vi "GUI_TapeDrive.vi"() -> ()   [LabVIEW 2013]
uses:
  Device Driver/TapeDrive/Mode_TypDEf.ctl
  Device Driver/shared/OnOffTypeDef.ctl
  shared programs/GUI_Template/GUI_master/tcp new data cluster.ctl
panel:
  in  "threshold_low::2":dbl=nan caption="threshold low" min=0.0 max=255.0
  in  "threshold_high::2":dbl=0.75 caption="threshold high" min=0.0 max=255.0
  in  "area_min::2":dbl=nan caption="min area" min=10.0 max=50000.0
  in  "area_max::2":dbl=0.75 caption="max area" min=10.0 max=50000.0
  out "cx::2":dbl=nan caption="x" min=0.0 max=0.0
  out "cy::2":dbl=nan caption="y" min=0.0 max=0.0
  out "oldpos::1":dbl=-887.082 caption="position" min=0.0 max=0.0
  out "try::1":dbl=2.0 caption="# of moves\n(scan mode)" min=0.0 max=0.0
  in  "fitnesslimit::2":dbl=0.75 caption="FitnessLimit" min=-100.0 max=1.0
  out "TapeOK":bool
  in  "exposure::3":dbl=0.01 caption="exposure" min=0.0001 max=1.0
  out "image::3":T1(plugin-control) caption="image"
  in  "GUIdevice 3":string="TapeMonitorCamTest"
  out "image::2":T1(plugin-control) caption="Monitor Image (binary)"
  out "particles::2":dbl=nan caption="particles" min=0.0 max=0.0
  out "symmetry::2":dbl=nan caption="Tape Monitor" min=0.0 max=0.0
  out "AreaSymmetry::2":dbl=nan caption="AreaSymmetry" min=0.0 max=0.0
  out "fitness::2":dbl=nan caption="fitness" min=0.0 max=0.0
  in  "TapeOK::2":T2 caption="TapeOK"
  in  "GUIdevice 2":string="TapeMonitorTest"
  in  "resetencoder::1":T2 caption="resetencoder"
  in  "TapeMotor::1":T2 caption="TapeDrive"
  in  "max velocity::1":dbl=5.0 caption="max velocity" min=1.0 max=2000.0
  in  "stepsize::1":dbl=2.0 caption="step size" min=1.0 max=100.0
  in  "timeout::1":dbl=500.0 caption="timeout" min=0.0 max=50000.0
  in  "Step::1":bool caption="Move Tape"
  out "pios chart":dbl(graph)=-887.082 caption="position"
  in  "redratio::1":dbl=1.0 caption="Ratio" min=-2.0 max=2.0
  in  "continious velocity::1":dbl=5.0 caption="continious velocity" min=1.0 max=100.0
  in  "velocity::1":dbl caption="velocity" min=0.0 max=0.0
  in  "Mode::1":T3 caption="Mode"
  in  "direction::1":bool=TRUE caption="Change direction"
  out "position::1":dbl=-887.082 caption="position" min=0.0 max=0.0
  in  "Test Cluster":T4
  out "device status::1":string="Initialized"
  in  "stop":bool
  in  "GUIdevice 1":string="TapeTest"
  # "4"
  # "1"
  # "TapeMotor"
  # "2"
  # "3"
  # "Symmetry"
  # "TapeMonitorCam"
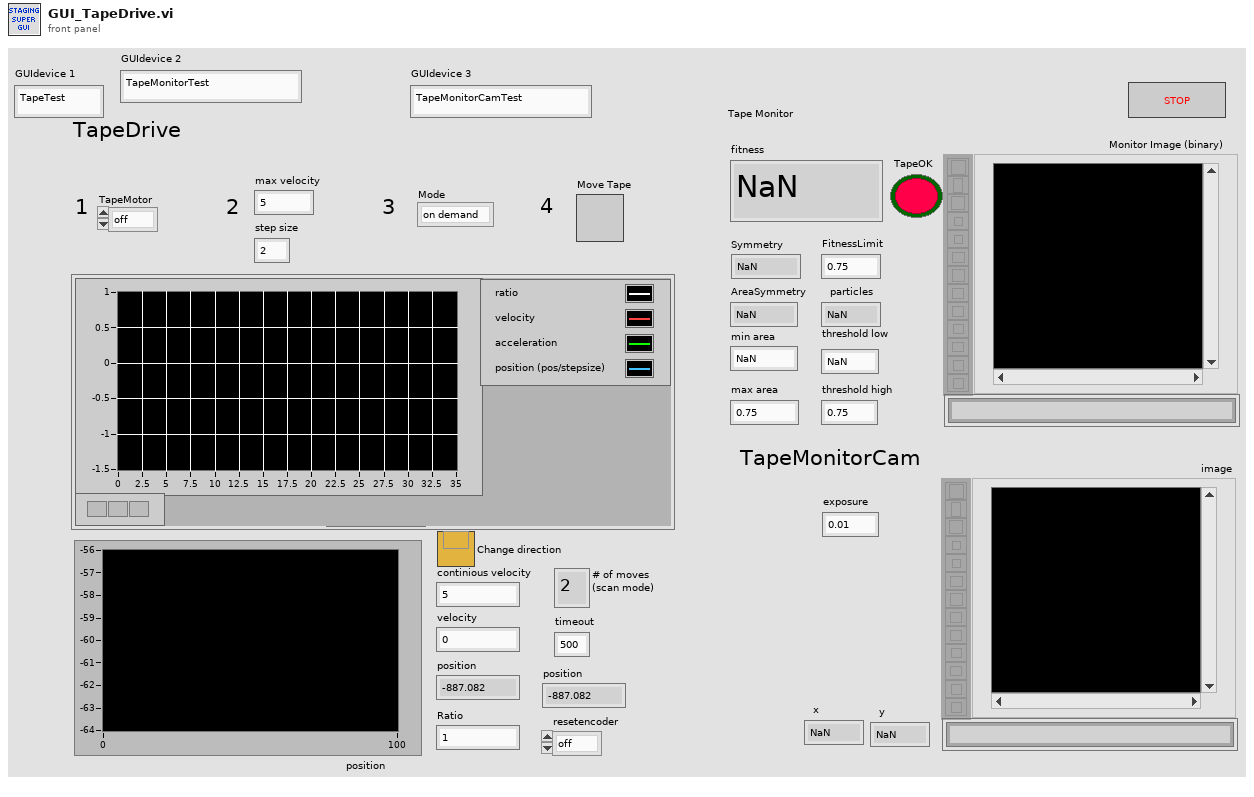
[diagram p1: front panel]
types:
  T1 = typedef "IMAQ Image.ctl" = refnum<image>
  T2 = typedef "OnOffTypeDef.ctl" = enum16{"off", "on"}
  T3 = typedef "Mode_TypDEf.ctl" = enum16{"on demand", "continuous", "scan"}
  T4 = cluster{"Channel::1":enum16{"Channel 0", "Channel 1", "Channel 2", "Channel 3"}, "Trajectory::1":waveform(dbl)[]}
  T5 = typedef "Image Type" = u32
  T6 = typedef "tcp new data cluster.ctl" = cluster{"EventEnum":enum16{"new data", "connection status update"}, "Device name":string}
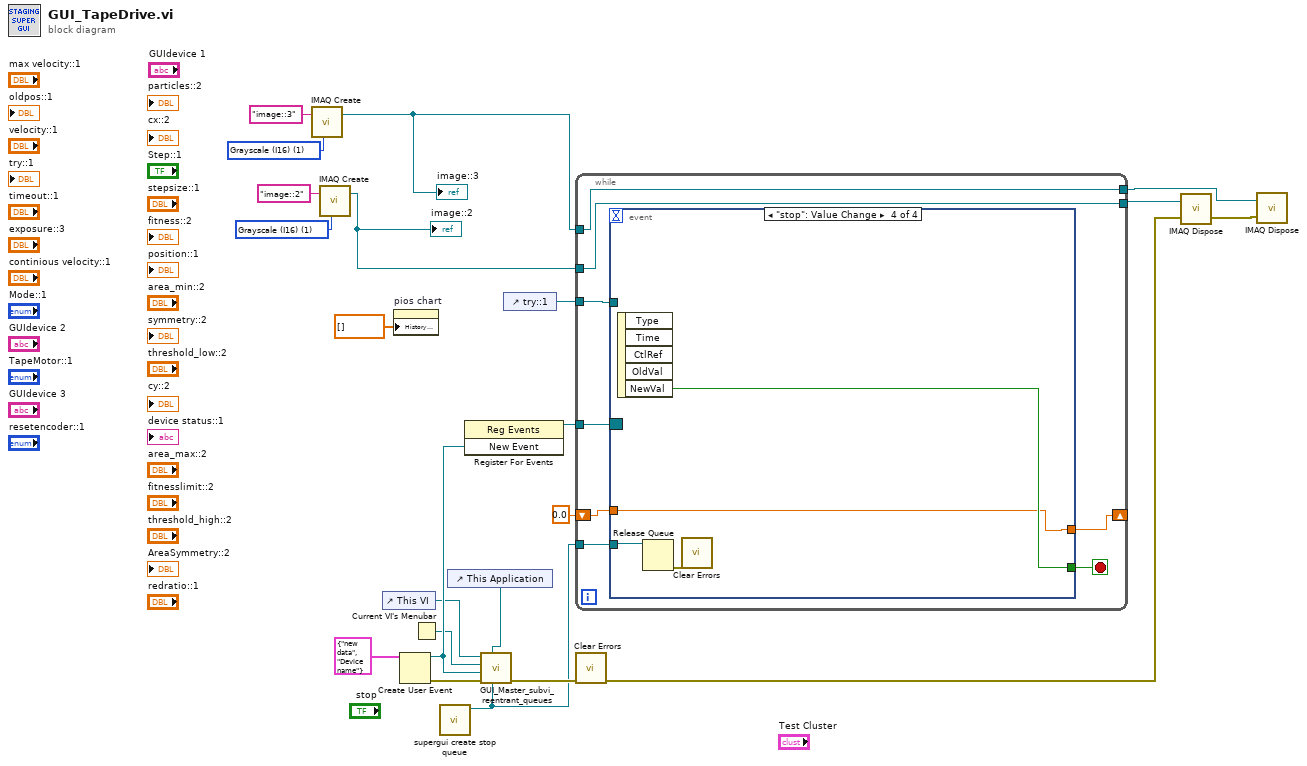
[diagram p0: block diagram]
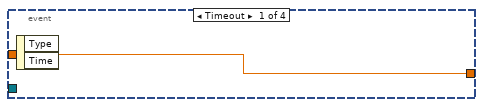
[diagram p2: hidden frame]
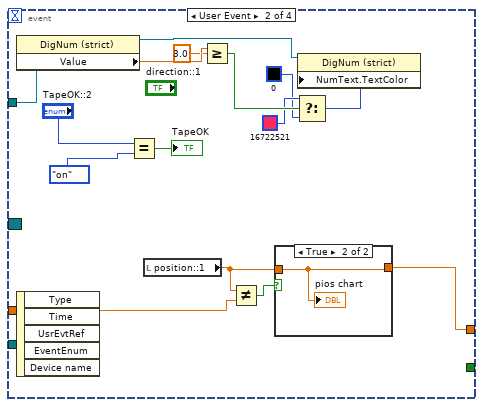
[diagram p3: hidden frame]
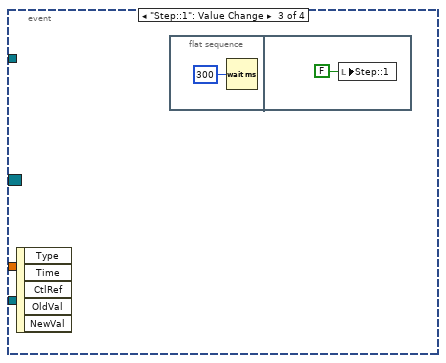
[diagram p5: hidden frame]
diagram:
  w10 = T5 1 items=["Grayscale (U8)", "Grayscale (I16)", "Grayscale (SGL)", "Complex (CSG)", "RGB (U32)", "HSL (U32)", "RGB (U64)", "Grayscale (U16)"] ("Image Type")
  w14 = T5 1 items=["Grayscale (U8)", "Grayscale (I16)", "Grayscale (SGL)", "Complex (CSG)", "RGB (U32)", "HSL (U32)", "RGB (U64)", "Grayscale (U16)"] ("Image Type")
  n1 = call "IMAQ Create"("Image Name"="image::3", "Image Type"=w10) -> ("New Image"=w8:T1)  [unwired: 3 in, 1 out]
  "image::3" <- w8
  n2 = call "IMAQ Create"("Image Name"="image::2", "Image Type"=w14) -> ("New Image"=w13:T1)  [unwired: 3 in, 1 out]
  "image::2" <- w13
  n3 = control-ref of="This VI"() -> (w4:refnum<vi>)
  n4 = property on="pios chart" class="WFChart (strict)"("History Data"=dbl[] []) -> ()  [unwired: 2 in, 2 out]
  n5 = Create User Event(user event datatype=T6 {"EventEnum"=enum."new data", "Device name"="Device name"} ("New Event")) -> (user event=w19:refnum<user-event>, error out=w21:errorcluster)  [unwired: 1 in]
  n6 = Current VI's Menubar() -> (w3:refnum<k9>)
  n7 = call "supergui create stop queue.vi"() -> ("STOP Queue out"=w1:refnum<queue>)  [unwired: 11 in]
  n8 = control-ref of="This Application"() -> (w2:refnum<vi>)
  n9 = register-events(w19) -> (reference out=w18:refnum<event-registration>)  [unwired: 2 in, 1 out]
  n10 = call "GUI_Master_subvi_reentrant_queues.vi"("STOP Queue in"=w1, "This Application"=w2, "error in (no error)"=w21, "tcp data event"=w19, "Caller menu reference"=w3, "Caller VI ref"=w4) -> ("error out"=w20:errorcluster)  [unwired: 5 in]
  n11 = control-ref of="try::1"() -> (w5:refnum<vi>)
  n12 = while {
    tunnel: w18 -> [w30]
    shift-right: [w27] -> _
    shift-left: 0.0 -> [w28]
    tunnel: w13 -> [w26]
    tunnel: [w26] -> w12
    tunnel: w8 -> [w25]
    tunnel: [w25] -> w6
    tunnel: w5 -> [w24]
    tunnel: w1 -> [w23]
    stop <- w29 stop-if-true
    n13 = event shown="[3] \"stop\": Value Change" {
      selector: w30 -> [_ _ _ _]
      dyn-events: _ -> [_ _ _ _]
      timeout: _ -> [_ _ _ _]
      tunnel: [_ _ _ w54] -> w29
      tunnel: w28 -> [w31 w46 _ w53]
      tunnel: [w31 w43 _ w53] -> w27
      tunnel: w24 -> [_ w39 _ _]
      tunnel: w23 -> [_ _ _ w52]
      event Timeout {
        n14 = event-data() -> ()  [unwired: 1 in, 2 out]
      }
      event User Event {
        n15 = property class="DigNum (strict)"(reference=w39) -> (reference out=w36:refnum<vi>, "Value"=w38:dbl)  [unwired: 1 in, 1 out]
        n16 = event-data() -> ()  [unwired: 1 in, 5 out]
        n17 = Equal?(x="TapeOK::2", y=OnOffTypeDef."on" ("TapeOK::2")) -> (x = y?=→"TapeOK":bool)
        n18 = local read "position::1"() -> (w44:dbl)
        n19 = Greater Or Equal?(x=w38, y=3.0) -> (x >= y?=w35:bool)
        n20 = Not Equal?(x=w44, y=w46) -> (x != y?=w45:bool)
        n21 = case shown="True" w45 {
          tunnel: w44 -> [w47 w48]
          tunnel: [w47 w48] -> w43
          frame False {
          }
          frame True {
            "pios chart" <- w48
          }
        }
        n22 = Select(t=u32 16722521, s=w35, f=u32 0) -> (s? t:f=w32:u32)
        n23 = property class="DigNum (strict)"(reference=w36, "NumText.TextColor"=w32) -> ()  [unwired: 1 in, 2 out]
      }
      event "Step::1": Value Change {
        n24 = event-data() -> ()  [unwired: 1 in, 5 out]
        n25 = flat-sequence {
          frame #0 {
            n26 = Wait (ms)(milliseconds to wait=u32 300) -> ()  [unwired: 1 out]
          }
          frame #1 {
            n27 = local write "Step::1"(FALSE ("Step::1")) -> ()
          }
        }
      }
      event "stop": Value Change {
        n28 = event-data() -> ("NewVal"=w54:bool)  [unwired: 1 in, 4 out]
        n29 = Release Queue(queue=w52) -> (error out=w51:errorcluster)  [unwired: 2 in, 2 out]
        n30 = call <vilib>:"Clear Errors.vi"("error in (no error)"=w51) -> ()  [unwired: 6 in, 1 out]
      }
    }
  }
  n31 = call <vilib>:"Clear Errors.vi"("error in (no error)"=w20) -> ("error out"=w11:errorcluster)  [unwired: 6 in]
  n32 = call "IMAQ Dispose"("Image"=w12, "error in (no error)"=w11) -> ("error out"=w7:errorcluster)  [unwired: 4 in]
  n33 = call "IMAQ Dispose"("Image"=w6, "error in (no error)"=w7) -> ()  [unwired: 4 in, 1 out]
